vi "AIsFIFORT-15-07-17.vi"(0 "FPGA VI Reference In":refnum<k20>, 1 "P2":dbl[](array[numeric]), 2 "P1":dbl[](array[numeric]), 3 "P0":dbl[](array[numeric]), 4 "error in":errorcluster) -> (5 "error out":errorcluster)   [LabVIEW 2010]
uses:
  <vilib>/rvi/interface/nirviMethod/nirviMethod.xnode
  C:/Users/HAGAR-IV/Desktop/Zeugs/markus/version feb 2012/FPGA Bitfiles/pertrasgcfpga2_FPGATarget_FPGA-Programm-05_A75D3647.lvbitx
  C:/Users/HAGAR-IV/Desktop/Zeugs/Johnny/pertrasgc fpga/FPGA-Programm-05-17.vi
  <vilib>/rvi/interface/common/niFpgaNodeNameForErrorReporting.ctl
  <vilib>/rvi/errors/niLvFpgaWhatHappensToTopLevelVI.ctl
  <vilib>/rvi/interface/nirviReadWriteControl/nirviReadWriteControl.xnode
  GVAIs.vi
  gvbooleschRT.vi
  <vilib>/Utility/error.llb/Error Cluster From Error Code.vi
  <vilib>/rvi/errors/niLvFpgaAdjustHostInterfaceError.vi
  NiFpgaLv.dll
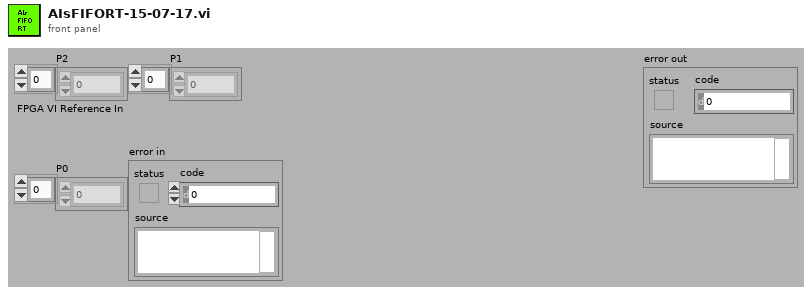
[diagram p1: front panel]
types:
  T1 = typedef "niFpgaNodeNameForErrorReporting.ctl" = enum16{"Open FPGA VI Reference", "Read/Write Control", "Invoke Method: Abort", "Invoke Method: Acknowledge IRQ", "Invoke Method: Download", "Invoke Method: FIFO.Configure", "Invoke Method: FIFO.Read", "Invoke Method: FIFO.Start", "Invoke Method: FIFO.Stop", "Invoke Method: FIFO.Write", "Invoke Method: Reset", "Invoke Method: Run", "Invoke Method: Wait on IRQ", "Close FPGA VI Reference"}
  T2 = typedef "niLvFpgaWhatHappensToTopLevelVI.ctl" = enum16{"top level VI scripted behind XNode", "top level VI inlined behind XNode"}
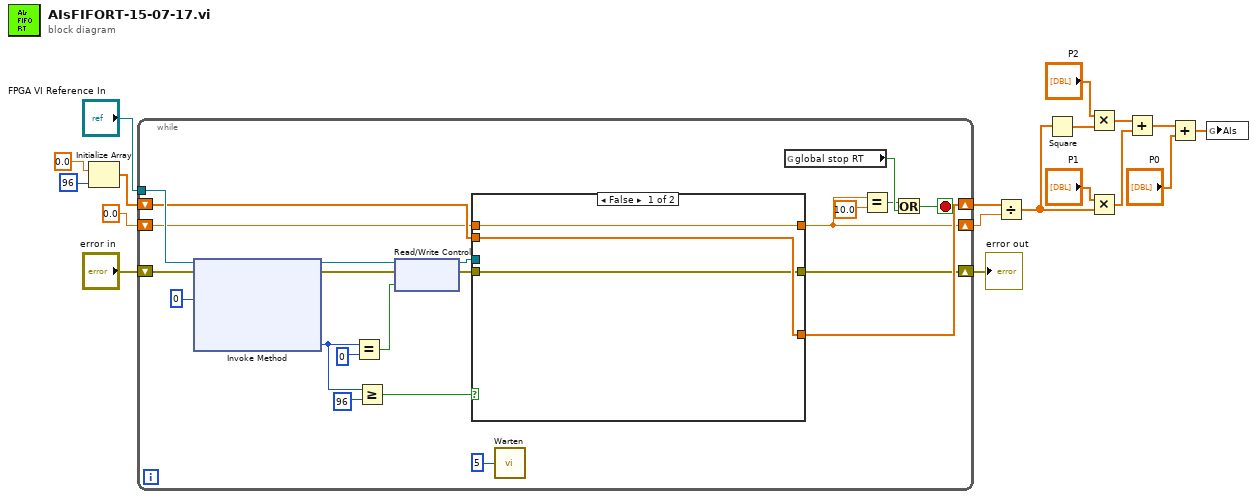
[diagram p0: block diagram]
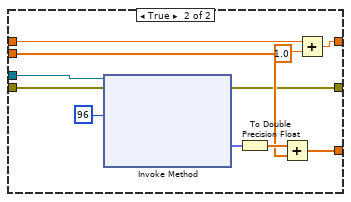
[diagram p2: hidden frame]
diagram:
  n1 = Initialize Array(0.0 ("Element"), 96 ("Dimension")) -> (w6:dbl[])
  n2 = while {
    tunnel: "FPGA VI Reference In" -> [w40]
    shift-right: [w34] -> w17
    shift-left: w6 -> [w35]
    shift-right: [w32] -> w5
    shift-left: 0.0 -> [w33]
    shift-right: [w19] -> w2
    shift-left: "error in" -> [w22]
    stop <- w25 stop-if-true
    n3 = xnode "Invoke Method"("FPGA VI Reference In"=w40, "error in"=w22, "Number of Elements"=u32 0) -> ("FPGA VI Reference Out"=w23:refnum<k20>, "error out"=w21:errorcluster, "Elements Remaining"=w30:u32)  [unwired: 1 in, 1 out]
    n4 = Equal?(x=w30, y=u32 0) -> (x = y?=w28:bool)
    n5 = Greater Or Equal?(x=w30, y=u32 96) -> (x >= y?=w37:bool)
    n6 = xnode "Read/Write Control"("FPGA VI Reference In"=w23, "error in"=w21, "FIFO leer"=w28) -> ("FPGA VI Reference Out"=w24:refnum<k20>, "error out"=w20:errorcluster)
    n7 = case shown="False" w37 {
      tunnel: w24 -> [_ w164]
      tunnel: w35 -> [w153 w160]
      tunnel: [w153 w159] -> w34
      tunnel: w33 -> [w152 w158]
      tunnel: [w152 w156] -> w32
      tunnel: w20 -> [w151 w155]
      tunnel: [w151 w154] -> w19
      frame False {
      }
      frame True {
        n8 = xnode "Invoke Method"("FPGA VI Reference In"=w164, "error in"=w155, "Number of Elements"=u32 96) -> ("error out"=w154:errorcluster, "Data"=w162:fxp<+/-,26,5>[])  [unwired: 1 in, 2 out]
        n9 = To Double Precision Float(number=w162) -> (double precision float=w161:dbl[])
        n10 = Add(x=w161, y=w160) -> (x+y=w159:dbl[])
        n11 = Add(x=w158, y=1.0) -> (x+y=w156:dbl)
      }
    }
    n12 = call "Warten"("Count(mSec)"=u32 5) -> ()  [unwired: 1 out]
    n13 = global read "gvbooleschRT.vi" "global stop RT"() -> (w27:bool)
    n14 = Equal?(x=w32, y=10.0) -> (x = y?=w26:bool)
    n15 = Or(x=w26, y=w27) -> (x .or. y?=w25:bool)
  }
  "error out" <- w2
  n16 = Divide(x=w17, y=w5) -> (x/y=w13:dbl[])
  n17 = Square(x=w13) -> (x^2=w16:dbl[])
  n18 = Multiply(x="P2", y=w16) -> (x*y=w12:dbl[])
  n19 = Multiply(x="P1", y=w13) -> (x*y=w11:dbl[])
  n20 = Add(x=w12, y=w11) -> (x+y=w10:dbl[])
  n21 = Add(x=w10, y="P0") -> (x+y=w4:dbl[])
  n22 = global write "GVAIs.vi" "AIs"(w4) -> ()
